vi "Load Rotator Modules.vi"(8 "Error In":errorcluster) -> (0 "Error Out":errorcluster, 2 "Menu control":T1, 3 "Modules":refnum<class "Template Module.lvclass">[](array[class]))   [LabVIEW 2018]
uses:
  LabActor/Template Module/Template Module.lvclass
  LabActor/Controllers/Application Controller/Menu Control.ctl
  LabActor/Instrument Actor/Instrument Actor.lvclass
  Users/arkady/Desktop/ado/github/LabActor/Template Module/Template Module.lvclass
  resonant_ultrasound_arxiv/maglab ultrasound -- arkady --arxiv/Stepper Controller/rotator driver.lvclass
  Users/arkady/Desktop/ado/github/NHMFL_Core/Libraries/Instruments/Instrument Driver/Instrument Driver.lvclass
  LabActor/Instrument Actor/Instrument Actor.lvclass/Instrument Actor.ctl
  LabActor/Template Module/Template Module.lvclass/Template Module.ctl
  LabActor/Template Module/Write Name.vi
  LabActor/Instrument Actor/Write Instrument driver.vi
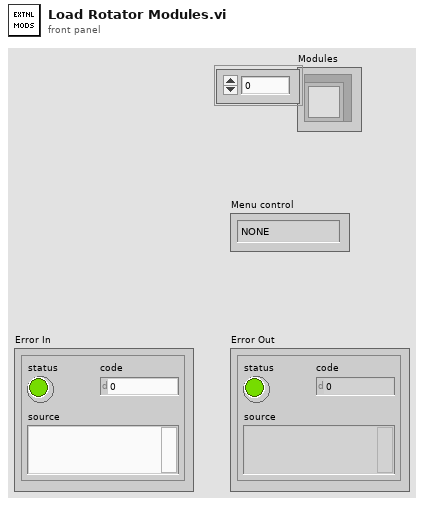
[diagram p1: front panel]
types:
  T1 = typedef "Menu Control.ctl" = enum16{"NONE", "Monitor", "Post-process", "Pulse"}
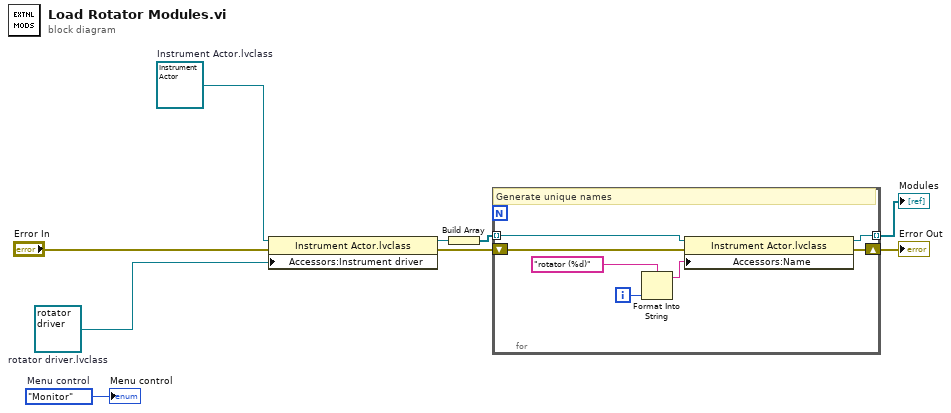
[diagram p0: block diagram]
diagram:
  w1 = refnum<class "rotator driver.lvclass"> refnum  # rotator driver.lvclass
  w7 = Menu_Control."Monitor"  # Menu control
  w9 = refnum<class "Instrument Actor.lvclass"> refnum  # Instrument Actor.lvclass
  n1 = property class="Instrument Actor.lvclass"(reference=w9, error in="Error In", "Accessors:Instrument driver"=w1) -> (reference out=w8:refnum<class "Instrument Actor.lvclass">, error out=w4:errorcluster)
  n2 = Build Array(w8) -> (w5:refnum<class "Instrument Actor.lvclass">[])
  n3 = for {
    tunnel: w5 -> [w16] mode=indexing
    shift-right: [w14] -> w2
    shift-left: w4 -> [w15]
    tunnel: [w13] -> w3 mode=indexing
    i -> [w12]
    # "Generate unique names"
    n4 = Format Into String(format string="rotator (%d)" ("Name"), w12) -> (resulting string=w10:string)  [unwired: 2 in, 1 out]
    n5 = property class="Instrument Actor.lvclass"(reference=w16, error in=w15, "Accessors:Name"=w10) -> (reference out=w13:refnum<class "Instrument Actor.lvclass">, error out=w14:errorcluster)
  }
  "Modules" <- w3
  "Error Out" <- w2
  "Menu control" <- w7
